vi "Test Tracker.vi"(7 "Command":string, 8 "error in (no error)":errorcluster, 9 "PPM":dbl format="%#_13g", 10 "Gas Name":string, 11 "Test Config":T1={"Chopper RPM"=140, "IR Power"=5, "Conc Tolerance"=0.0, "Gas Stable Time"=0, "A-D Settle"=0, "Samples"=0, "Filter Time"=0, "Gas Mixtures"=[], "Filter Sequences"=[], "Functional Test"={"Mic Test ON ADC Max"=0.0, "Mic Test ON ADC Min"=0.0, "Mic Test OFF ADC Max"=0.0, "Mic Test OFF ADC Min"=0.0, "Mic Test IC ADC Max"=0.0, "Mic Test IC ADC Min"=0.0, "IR Emitter ON ADC Max"=0.0, "IR Emitter ON ADC Min"=0.0, "IR Emitter OFF ADC Max"=0.0, "IR Emitter OFF ADC Min"=0.0}, "Initial Flow Rate"=0.0, "Max Flow Rate"=0.0} {"Gas Mixtures"."ADC Gains" items=["0"=0, "3"=3, "4"=4, "5"=5, "6"=6, "7"=7]; "Conc Tolerance" min=0.0 max=100.0 step=1.0; "IR Power" min=2 max=5 step=1; "Chopper RPM" min=140 max=1000 step=1}) -> (0 "error out":errorcluster, 2 "Gas Index":i32, 3 "Proceed?":bool, 5 "All Done?":bool)   [LabVIEW 2015]
uses:
  Controls/Test Config.ctl
  Controls/Gas Mixture.ctl
  CAN Communication/PAS/Typedefs/ADC Gains.ctl
  Controls/Filter Sequence.ctl
  Controls/Functional Test.ctl
  CAN Communication/PAS/PAS.lvclass
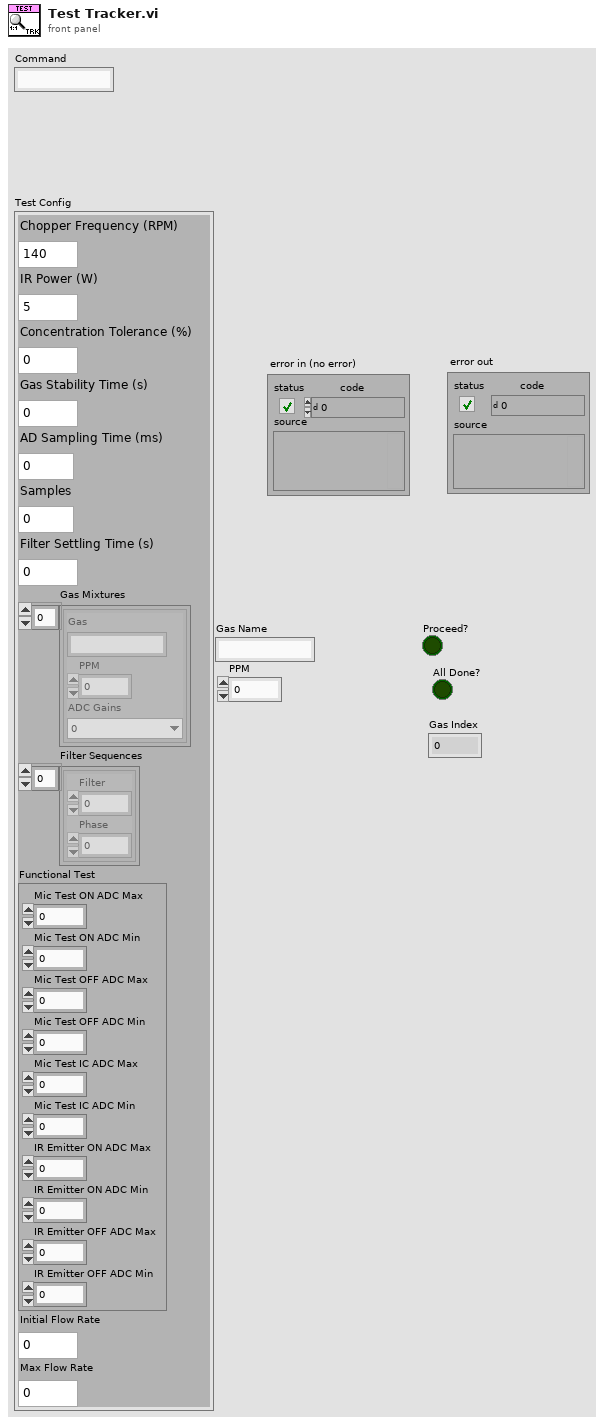
[diagram p1: front panel]
types:
  T1 = typedef "Test Config.ctl" = cluster{"Chopper RPM":u16, "IR Power":u8, "Conc Tolerance":dbl, "Gas Stable Time":u16, "A-D Settle":u16, "Samples":u16, "Filter Time":u16, "Gas Mixtures":T2[], "Filter Sequences":T4[], "Functional Test":T5, "Initial Flow Rate":sgl, "Max Flow Rate":sgl}
  T2 = typedef "Gas Mixture.ctl" = cluster{"Gas":string, "PPM":dbl, "ADC Gains":T3}
  T3 = typedef "PAS.lvclass/ADC Gains.ctl" = u16
  T4 = typedef "Filter Sequence.ctl" = cluster{"Filter":u8, "Phase":dbl}
  T5 = typedef "Functional Test.ctl" = cluster{"Mic Test ON ADC Max":dbl, "Mic Test ON ADC Min":dbl, "Mic Test OFF ADC Max":dbl, "Mic Test OFF ADC Min":dbl, "Mic Test IC ADC Max":dbl, "Mic Test IC ADC Min":dbl, "IR Emitter ON ADC Max":dbl, "IR Emitter ON ADC Min":dbl, "IR Emitter OFF ADC Max":dbl, "IR Emitter OFF ADC Min":dbl}
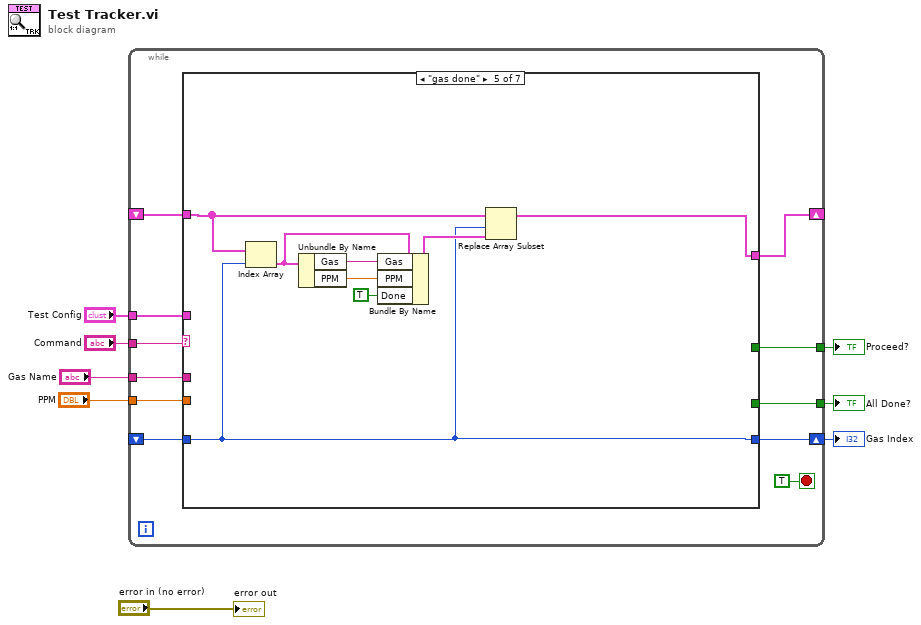
[diagram p0: block diagram]
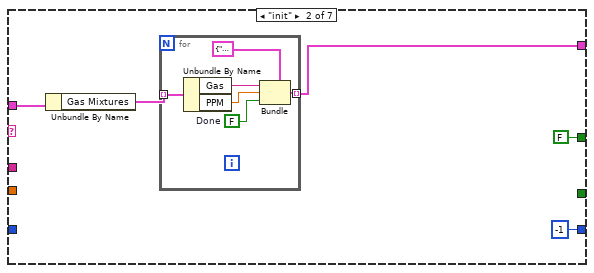
[diagram p3: hidden frame]
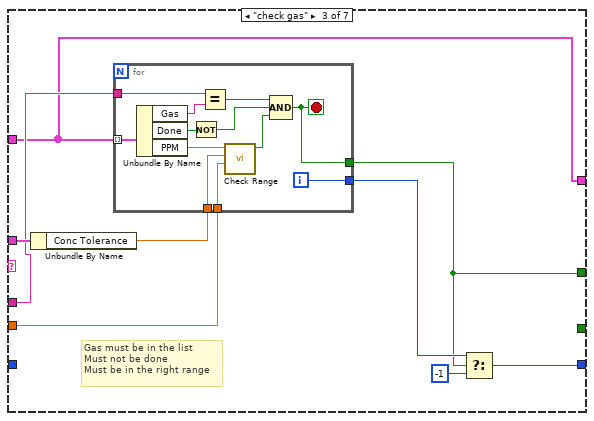
[diagram p4: hidden frame]
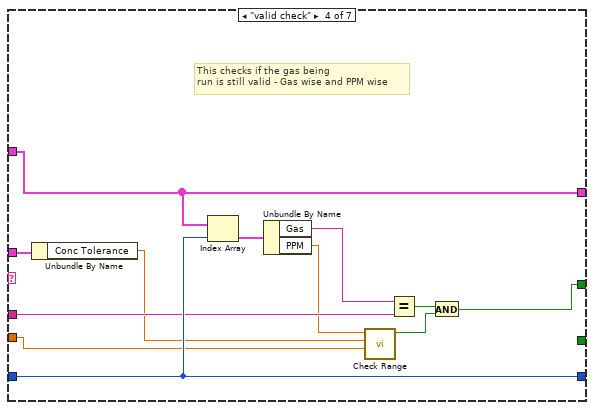
[diagram p5: hidden frame]
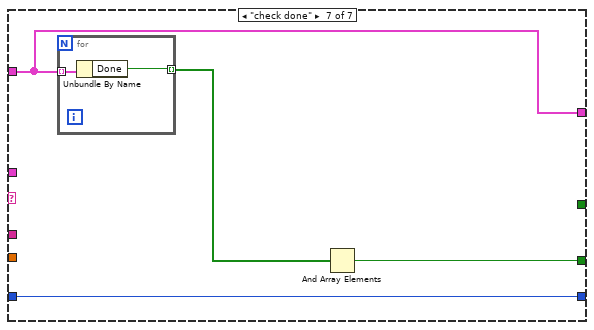
[diagram p7: hidden frame]
diagram:
  n1 = while {
    tunnel: "Command" -> [w19]
    shift-right: [w17] -> _
    shift-left: _ -> [w16]
    tunnel: "Gas Name" -> [w14]
    tunnel: "PPM" -> [w13]
    tunnel: [w12] -> w3
    shift-right: [w11] -> w2
    shift-left: _ -> [w9]
    tunnel: [w10] -> w1
    tunnel: "Test Config" -> [w15]
    stop <- TRUE stop-if-true
    n2 = case shown="\"gas done\"" w19 {
      tunnel: w15 -> [_ w26 w41 w59 _ _ _]
      tunnel: [w21 w22 w34 w65 w73 w74 w76] -> w17
      tunnel: w16 -> [w21 _ w34 w65 w72 w74 w76]
      tunnel: w14 -> [_ _ w37 w61 _ _ _]
      tunnel: w13 -> [_ _ w38 w60 _ _ _]
      tunnel: [_ FALSE w33 w54 _ _ _] -> w12
      tunnel: [w20 -1 ("index of element") w40 w64 w66 w75 w78] -> w11
      tunnel: [_ _ _ _ _ _ w79] -> w10
      tunnel: w9 -> [w20 _ _ w64 w66 w75 w78]
      frame Default {
      }
      frame "init" {
        n3 = Unbundle By Name(w26) -> ("Gas Mixtures"=w25:T2[])
        n4 = for {
          tunnel: w25 -> [w32] mode=indexing
          tunnel: [w27] -> w22 mode=indexing
          w29 = FALSE  # Done
          n5 = Unbundle By Name(w32) -> ("Gas"=w31:string, "PPM"=w30:dbl)
          n6 = Bundle(cluster=cluster{"Gas":string, "PPM":dbl, "Done":bool} {"Gas"="", "PPM"=0.0, "Done"=FALSE}, "Gas"=w31, "PPM"=w30, "Done"=w29) -> (w27:cluster{"Gas":string, "PPM":dbl, "Done":bool})
        }
      }
      frame "check gas" {
        # "Gas must be in the list\nMust not be done\nMust be in the right range"
        n7 = Unbundle By Name(w41) -> ("Conc Tolerance"=w39:dbl)
        n8 = for {
          tunnel: w34 -> [w53] mode=indexing
          tunnel: w39 -> [w51]
          tunnel: w38 -> [w50]
          tunnel: w37 -> [w49]
          tunnel: [w43] -> w33
          tunnel: [w42] -> w35
          i -> [w42]
          stop <- w43 stop-if-true
          n9 = Unbundle By Name(w53) -> ("Gas"=w48:string, "Done"=w45:bool, "PPM"=w52:dbl)
          n10 = Not(x=w45) -> (.not. x?=w44:bool)
          n11 = Equal?(x=w49, y=w48) -> (x = y?=w47:bool)
          n12 = call "Check Range.vi"("Actual PPM"=w50, "Tolerance"=w51, "PPM Spec"=w52) -> ("In Range?"=w46:bool)  [unwired: 7 in, 1 out]
          n13 = Compound Arithmetic op=AND(w47, w44, w46) -> (w43:bool)
        }
        n14 = Select(t=w35, s=w33, f=-1 ("index of element")) -> (s? t:f=w40:i32)
      }
      frame "valid check" {
        # "This checks if the gas being\nrun is still valid - Gas wise and PPM wise"
        n15 = Unbundle By Name(w59) -> ("Conc Tolerance"=w58:dbl)
        n16 = Index Array(array=w65, index=w64) -> (element=w63:cluster{"Gas":string, "PPM":dbl, "Done":bool})
        n17 = Unbundle By Name(w63) -> ("Gas"=w62:string, "PPM"=w57:dbl)
        n18 = call "Check Range.vi"("Actual PPM"=w60, "Tolerance"=w58, "PPM Spec"=w57) -> ("In Range?"=w55:bool)  [unwired: 7 in, 1 out]
        n19 = Equal?(x=w62, y=w61) -> (x = y?=w56:bool)
        n20 = And(x=w56, y=w55) -> (x .and. y?=w54:bool)
      }
      frame "gas done" {
        n21 = Index Array(array=w72, index=w66) -> (element=w70:cluster{"Gas":string, "PPM":dbl, "Done":bool})
        n22 = Unbundle By Name(w70) -> ("Gas"=w71:string, "PPM"=w69:dbl)
        n23 = Bundle By Name(cluster=w70, "Gas"=w71, "PPM"=w69, "Done"=TRUE) -> (w67:cluster{"Gas":string, "PPM":dbl, "Done":bool})
        n24 = Replace Array Subset(array=w72, new element=w67, index=w66) -> (w73:cluster{"Gas":string, "PPM":dbl, "Done":bool}[])
      }
      frame "get gas" {
      }
      frame "check done" {
        n25 = for {
          tunnel: w76 -> [w81] mode=indexing
          tunnel: [w80] -> w77 mode=indexing
          n26 = Unbundle By Name(w81) -> ("Done"=w80:bool)
        }
        n27 = And Array Elements(Boolean array=w77) -> (logical AND=w79:bool)
      }
    }
  }
  "Proceed?" <- w3
  "Gas Index" <- w2
  "All Done?" <- w1
  "error out" <- "error in (no error)"
